vi "MIC_MD.vi"() -> ()   [LabVIEW 2012]
uses:
  GFG/GFGfpRefGet.vi
  GFG/GFGnumericGet.vi
  GFG/GFG library.lvlib
panel:
  out "Source VI":string
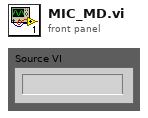
[diagram p1: front panel]
types:
  T1 = enum8{"Enabled", "Disabled", "Disabled and Grayed Out"}
  T2 = cluster{"WaveformChartRef":refnum<vi>, "DigitalRef":refnum<vi>, "ArrayRef":refnum<vi>, "TabControlRef":refnum<vi>, "EnumRef":refnum<vi>, "RingRef":refnum<vi>, "BooleanRef":refnum<vi>, "KnobRef":refnum<vi>, "SlideRef":refnum<vi>, "PathRef":refnum<vi>, "StringRef":refnum<vi>, "ComboBox":refnum<vi>, "WaveformGraphRef":refnum<vi>}
  T3 = enum16{"Left Button", "Center Button", "Right Button", "Window Close"}
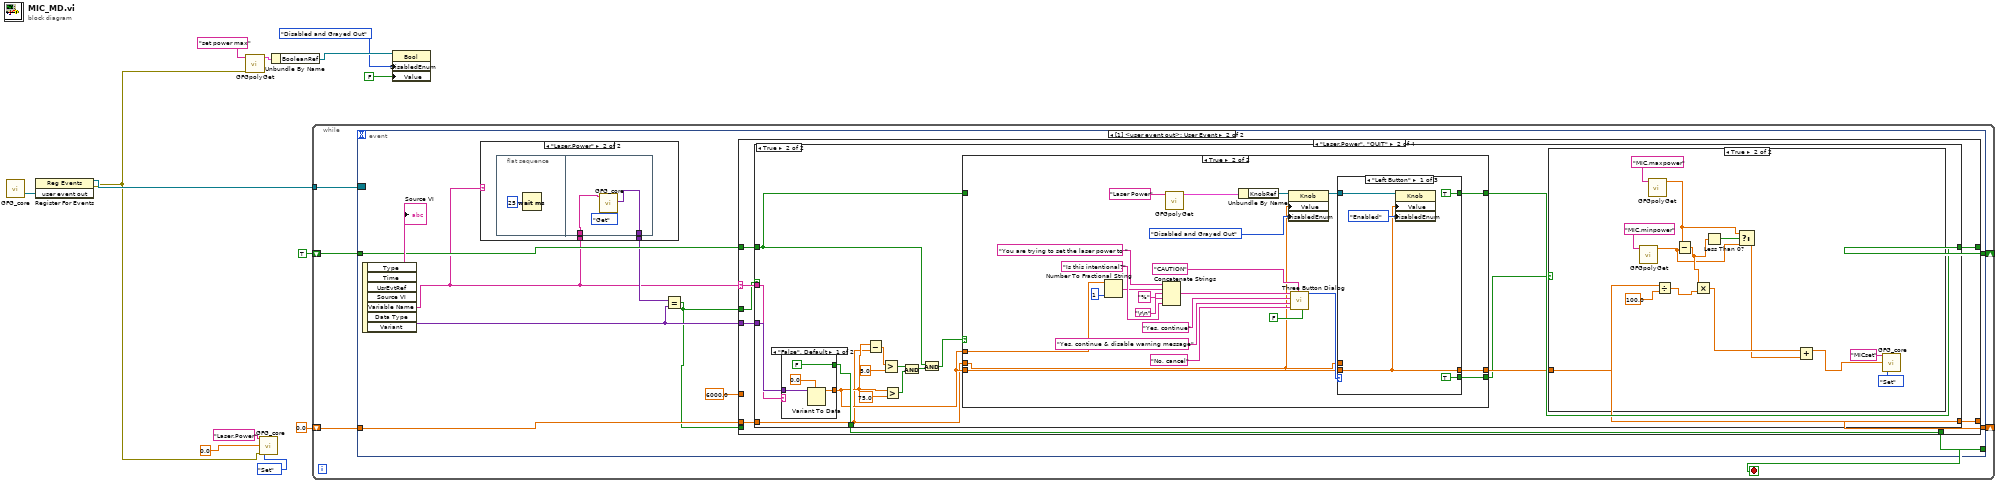
[diagram p0: block diagram]
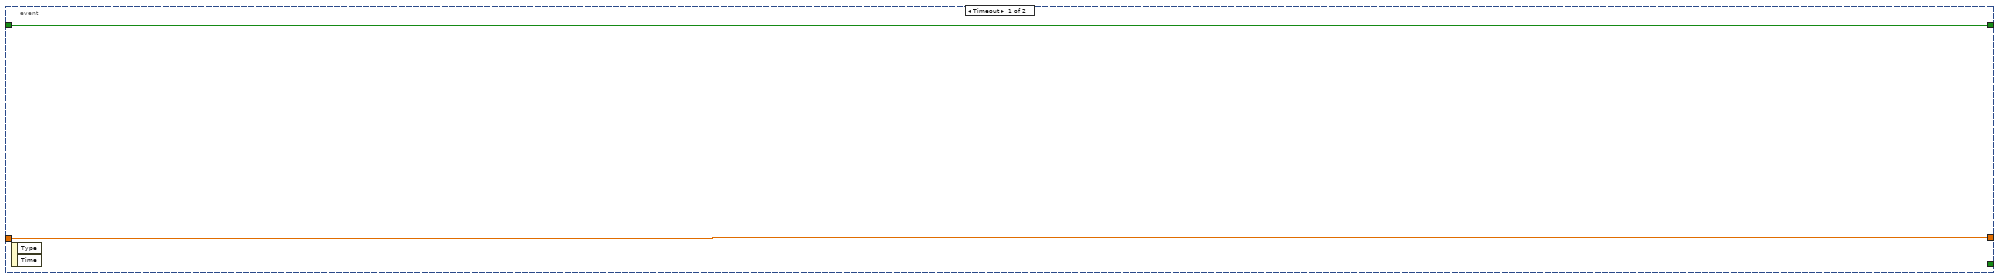
[diagram p2: hidden frame]
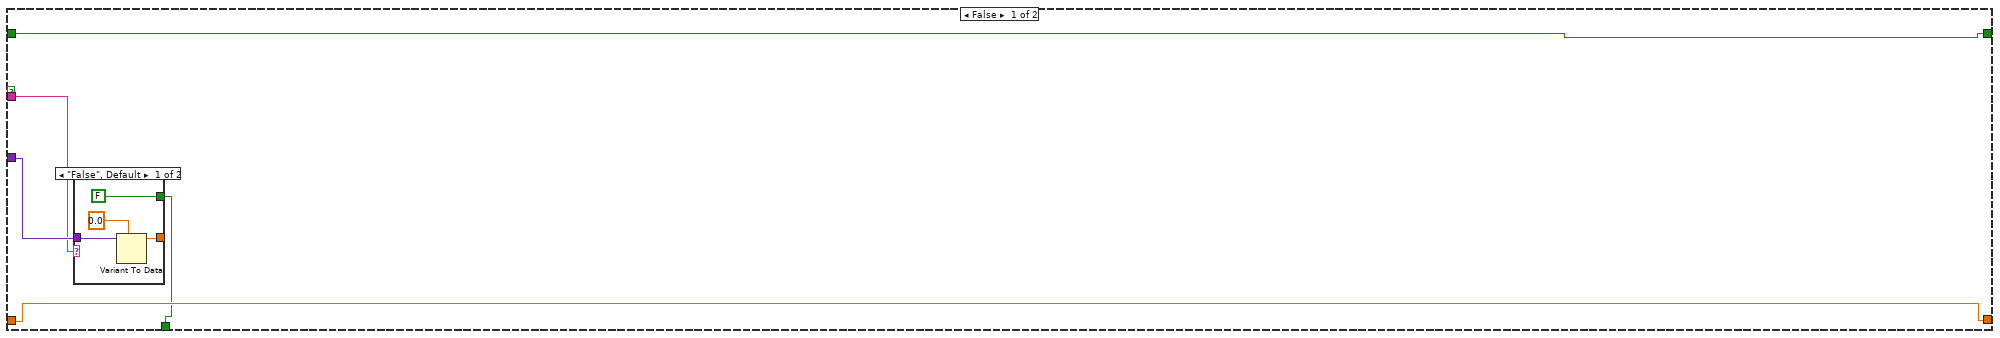
[diagram p5: hidden frame]
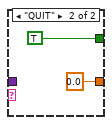
[diagram p6: hidden frame]
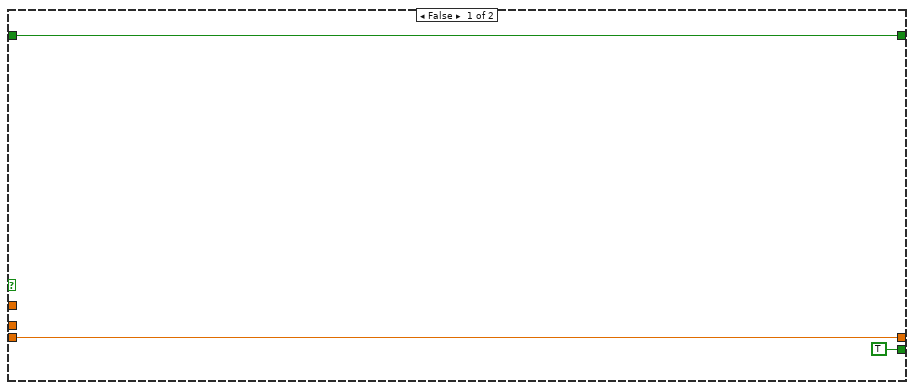
[diagram p8: hidden frame]
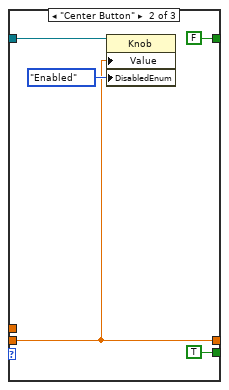
[diagram p9: hidden frame]
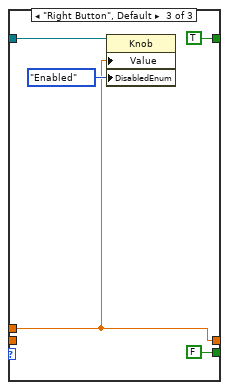
[diagram p10: hidden frame]
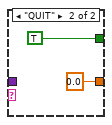
[diagram p11: hidden frame]
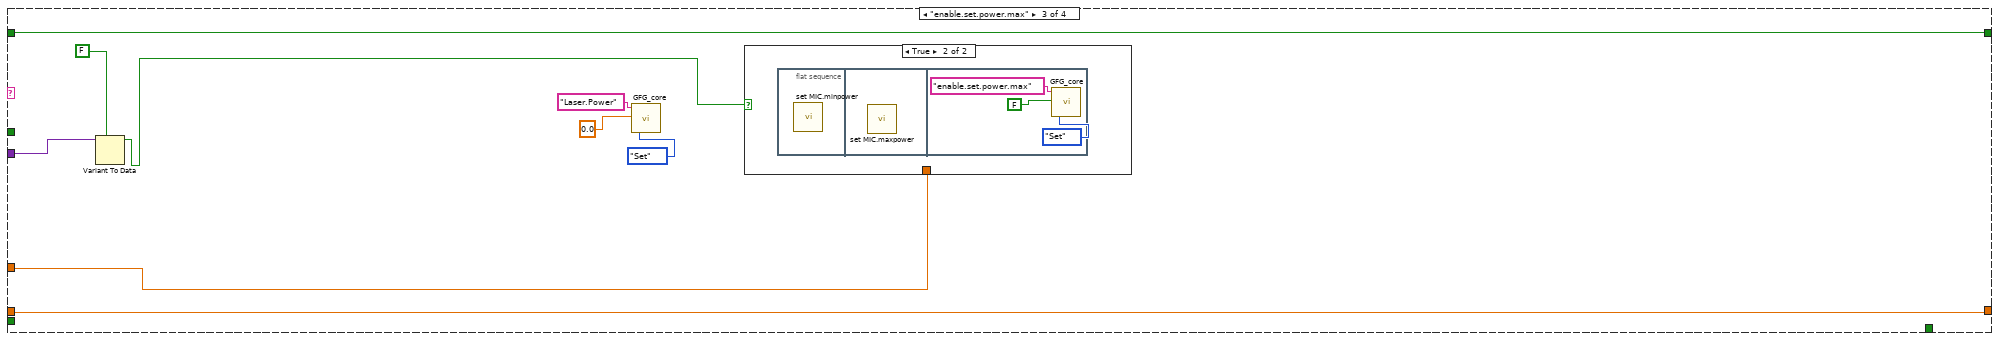
[diagram p12: hidden frame]
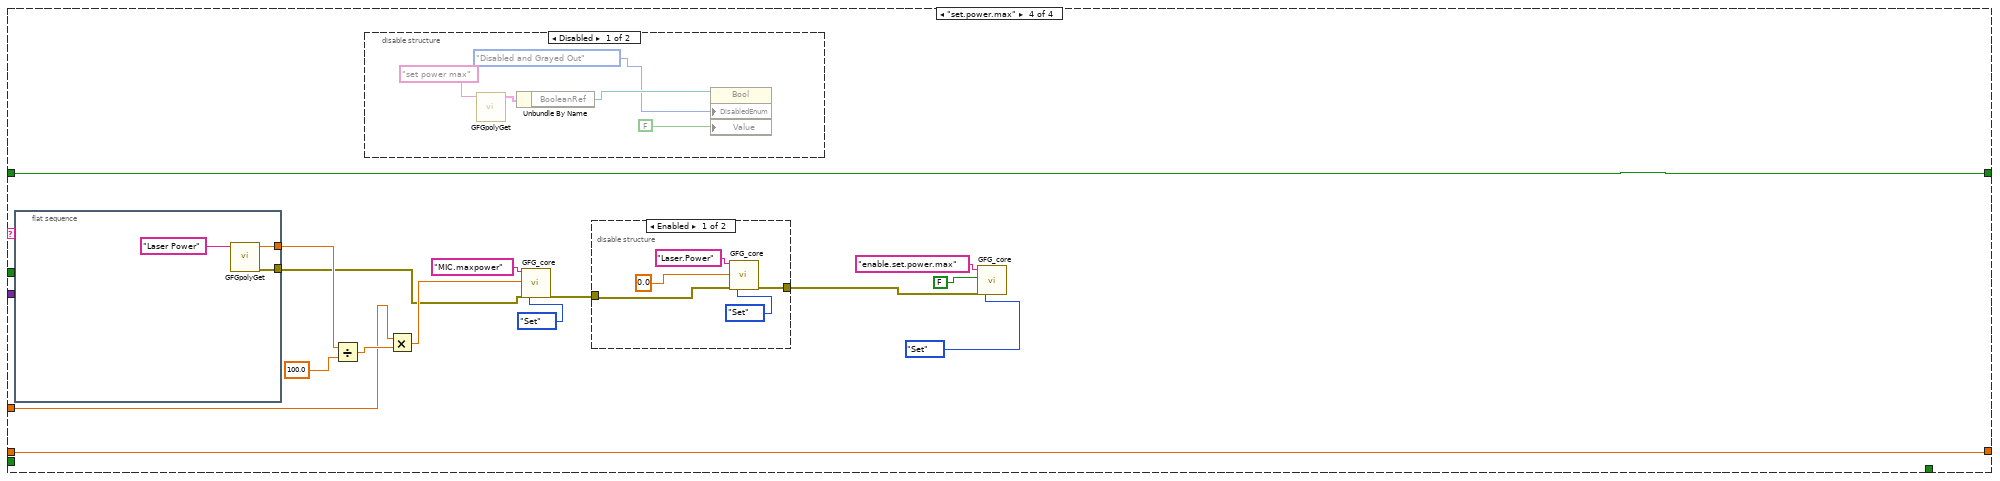
[diagram p14: hidden frame]
diagram:
  n1 = call "GFG_core.vi"() -> ("user event out"=w13:refnum<user-event>)  [unwired: 13 in, 6 out]
  n2 = register-events(w13) -> (reference out=w12:refnum<event-registration>, error out=w1:errorcluster)  [unwired: 2 in]
  n3 = call-poly "GFGpolyGet.vi"("error in (no error)"=w1, "Variable Name in"="set power max") -> ("output cluster"=w4:T2)  [unwired: 8 in, 1 out]
  n4 = call "GFG_core.vi"("Variable Name in"="Laser.Power", "Variant in"=0.0 ("Laser Power"), "error in (no error)"=w1, "Action"=enum16{"Init", "Set", "Get"}."Set") -> ()  [unwired: 9 in, 7 out]
  n5 = Unbundle By Name(w4) -> ("BooleanRef"=w5:refnum<vi>)
  n6 = while {
    tunnel: w12 -> [w19]
    shift-right: [w17] -> _
    shift-left: 0.0 ("Laser Power") -> [w16]
    shift-right: [w15] -> _
    shift-left: TRUE -> [w14]
    stop <- w18 stop-if-true
    n7 = event shown="[1] <user event out>: User Event" {
      selector: w19 -> [_ _]
      dyn-events: _ -> [_ _]
      timeout: _ -> [_ _]
      tunnel: [_ w31] -> w18
      tunnel: [w21 w30] -> w17
      tunnel: w16 -> [w21 w29]
      tunnel: [w20 w28] -> w15
      tunnel: w14 -> [w20 w27]
      event Timeout {
        n8 = event-data() -> ()  [unwired: 1 in, 2 out]
      }
      event User Event {
        n9 = event-data() -> ("Source VI"=→"Source VI":string, "Variable Name"=w22:string, "Variant"=w25:variant)  [unwired: 1 in, 4 out]
        n10 = case shown="\"Laser.Power\"" w22 {
          tunnel: w22 -> [w33 w35]
          tunnel: [w33 w34] -> w24
          frame "False", Default {
          }
          frame "Laser.Power" {
            n11 = flat-sequence {
              tunnel: w35 -> [w38]
              tunnel: [w37] -> w34
              frame #0 {
                n12 = Wait (ms)(milliseconds to wait=u32 25) -> ()  [unwired: 1 out]
              }
              frame #1 {
                n13 = call "GFG_core.vi"("Variable Name in"=w38, "Action"=enum16{"Init", "Set", "Get"}."Get") -> ("Variant Out"=w37:variant)  [unwired: 11 in, 6 out]
              }
            }
          }
        }
        n14 = Equal?(x=w24, y=w25) -> (x = y?=w23:bool)
        n15 = case shown="\"Laser.Power\", \"QUIT\"" w22 {
          selector: w22 -> [_ w48 _ _]
          tunnel: w25 -> [_ w49 w142 _]
          tunnel: [_ w47 _ _] -> w31
          tunnel: [w41 w44 w147 w165] -> w30
          tunnel: w29 -> [w41 w43 w147 w165]
          tunnel: [w40 w46 w146 w164] -> w28
          tunnel: w27 -> [w40 w45 w146 w164]
          tunnel: 6000.0 ("Laser Power") -> [_ _ w139 w151]
          tunnel: w23 -> [_ _ _ _]
          tunnel: w23 -> [_ w42 _ _]
          frame "False", Default {
          }
          frame "Laser.Power", "QUIT" {
            n16 = case shown="True" w42 {
              tunnel: w49 -> [w52 w76]
              tunnel: w48 -> [w51 w75]
              tunnel: [w50 w74] -> w47
              tunnel: [w53 w71] -> w46
              tunnel: w45 -> [w53 w69]
              tunnel: [w54 w68] -> w44
              tunnel: w43 -> [w54 w65]
              frame False {
                n17 = case shown="\"False\", Default" w51 {
                  tunnel: w52 -> [w58 _]
                  tunnel: [w57 0.0 ("Laser Power")] -> _
                  tunnel: [FALSE TRUE] -> w50
                  frame "False", Default {
                    n18 = Variant To Data(type=0.0 ("Laser Power"), Variant=w58) -> (data=w57:dbl)  [unwired: 1 in, 1 out]
                  }
                  frame "QUIT" {
                  }
                }
              }
              frame True {
                n19 = case shown="\"False\", Default" w75 {
                  tunnel: w76 -> [w136 _]
                  tunnel: [w135 0.0 ("Laser Power")] -> w66
                  tunnel: [FALSE TRUE] -> w74
                  frame "False", Default {
                    n20 = Variant To Data(type=0.0 ("Laser Power"), Variant=w136) -> (data=w135:dbl)  [unwired: 1 in, 1 out]
                  }
                  frame "QUIT" {
                  }
                }
                n21 = Subtract(x=w66, y=w65) -> (x-y=w64:dbl)
                n22 = Greater?(x=w64, y=5.0) -> (0:w62:bool)
                n23 = Greater?(x=w66, y=75.0) -> (0:w73:bool)
                n24 = And(x=w62, y=w73) -> (x .and. y?=w67:bool)
                n25 = And(x=w69, y=w67) -> (x .and. y?=w70:bool)
                n26 = case shown="True" w70 {
                  tunnel: [TRUE w111] -> w61
                  tunnel: [w92 w110] -> w71
                  tunnel: w69 -> [w92 _]
                  tunnel: w65 -> [_ w98]
                  tunnel: w66 -> [_ w108]
                  tunnel: w66 -> [w91 w99]
                  tunnel: [w91 w94] -> w68
                  frame False {
                  }
                  frame True {
                    n27 = Number To Fractional String(number=w108, precision (6)=i16 1) -> (F-format string=w97:string)  [unwired: 2 in]
                    n28 = Concatenate Strings("You are trying to set the laser power to " ("message"), w97, "%" ("string"), "\r\n", "Is this intentional?" ("string")) -> (w105:string)
                    n29 = call-poly "GFGpolyGet.vi"("Variable Name in"="Laser Power") -> ("output cluster"=w103:T2)  [unwired: 9 in, 1 out]
                    n30 = Unbundle By Name(w103) -> ("KnobRef"=w102:refnum<vi>)
                    n31 = property class="Knob"(reference=w102, "Value"=w98, "DisabledEnum"=T1."Disabled and Grayed Out" ("Disabled")) -> (reference out=w100:refnum<vi>)  [unwired: 1 in, 1 out]
                    n32 = call <vilib>:"Three Button Dialog.vi"("Allow user to close window? (TRUE)"=FALSE, "Window Title (\"\")"="CAUTION" ("Window Title (\"\")"), "Right Button Text (\"Cancel\")"="No, cancel" ("Right Button Text (\"Cancel\")"), "Center Button Text (\"No\")"="Yes, continue & disable warning message" ("Center Button Text (\"No\")"), "Left Button Text (\"Yes\")"="Yes, continue" ("Left Button Text (\"Yes\")"), "message"=w105) -> ("Which Button?"=w112:T3)  [unwired: 5 in]
                    n33 = case shown="\"Left Button\"" w112 {
                      tunnel: [TRUE TRUE FALSE] -> w111
                      tunnel: [TRUE FALSE TRUE] -> w110
                      tunnel: w100 -> [w119 w124 w129]
                      tunnel: w99 -> [w118 w123 _]
                      tunnel: w98 -> [_ _ w128]
                      tunnel: [w118 w123 w128] -> w94
                      frame "Left Button" {
                        n34 = property class="Knob"(reference=w119, "Value"=w118, "DisabledEnum"=T1."Enabled" ("Disabled")) -> ()  [unwired: 1 in, 2 out]
                      }
                      frame "Center Button" {
                        n35 = property class="Knob"(reference=w124, "Value"=w123, "DisabledEnum"=T1."Enabled" ("Disabled")) -> ()  [unwired: 1 in, 2 out]
                      }
                      frame "Right Button", Default {
                        n36 = property class="Knob"(reference=w129, "Value"=w128, "DisabledEnum"=T1."Enabled" ("Disabled")) -> ()  [unwired: 1 in, 2 out]
                      }
                    }
                  }
                }
                n37 = case shown="True" w61 {
                  tunnel: w68 -> [_ w87]
                  frame False {
                  }
                  frame True {
                    n38 = call-poly "GFGpolyGet.vi"("Variable Name in"="MIC.minpower") -> ("Numeric"=w79:dbl)  [unwired: 9 in, 1 out]
                    n39 = call-poly "GFGpolyGet.vi"("Variable Name in"="MIC.maxpower") -> ("Numeric"=w82:dbl)  [unwired: 9 in, 1 out]
                    n40 = Divide(x=w87, y=100.0 ("x")) -> (x/y=w90:dbl)
                    n41 = Subtract(x=w82, y=w79) -> (x-y=w84:dbl)
                    n42 = Multiply(x=w84, y=w90) -> (x*y=w88:dbl)
                    n43 = Less Than 0?(x=w84) -> (x < 0?=w83:bool)
                    n44 = Select(t=w82, s=w83, f=w79) -> (s? t:f=w80:dbl)
                    n45 = Add(x=w88, y=w80) -> (x+y=w81:dbl)
                    n46 = call "GFG_core.vi"("Variable Name in"="MICset", "Variant in"=w81, "Action"=enum16{"Init", "Set", "Get"}."Set") -> ()  [unwired: 10 in, 7 out]
                  }
                }
              }
            }
          }
          frame "enable.set.power.max" {
            n47 = Variant To Data(type=FALSE, Variant=w142) -> (data=w140:bool)  [unwired: 1 in, 1 out]
            n48 = call "GFG_core.vi"("Variable Name in"="Laser.Power", "Variant in"=0.0 ("Laser Power"), "Action"=enum16{"Init", "Set", "Get"}."Set") -> ()  [unwired: 10 in, 7 out]
            n49 = case shown="True" w140 {
              tunnel: w139 -> [_ _]
              frame False {
              }
              frame True {
                n50 = flat-sequence {
                  frame #0 {
                    n51 = call "set MIC.minpower.vi"() -> ()  [unwired: 12 in]
                  }
                  frame #1 {
                    n52 = call "set MIC.maxpower.vi"() -> ()  [unwired: 12 in]
                  }
                  frame #2 {
                    n53 = call "GFG_core.vi"("Variable Name in"="enable.set.power.max", "Variant in"=FALSE, "Action"=enum16{"Init", "Set", "Get"}."Set") -> ()  [unwired: 10 in, 7 out]
                  }
                }
              }
            }
          }
          frame "set.power.max" {
            n54 = flat-sequence {
              tunnel: [w172] -> w160
              tunnel: [w171] -> w157
              frame #0 {
                n55 = call-poly "GFGpolyGet.vi"("Variable Name in"="Laser Power") -> ("error out"=w171:errorcluster, "Numeric"=w172:dbl)  [unwired: 9 in]
              }
            }
            n56 = Divide(x=w160, y=100.0 ("x")) -> (x/y=w159:dbl)
            n57 = disable-structure shown="Disabled" {
              frame Disabled {
                n58 = call-poly "GFGpolyGet.vi"("Variable Name in"="set power max") -> ("output cluster"=w177:T2)  [unwired: 9 in, 1 out]
                n59 = Unbundle By Name(w177) -> ("BooleanRef"=w176:refnum<vi>)
                n60 = property class="Bool"(reference=w176, "DisabledEnum"=T1."Disabled and Grayed Out" ("Disabled"), "Value"=FALSE) -> ()  [unwired: 1 in, 2 out]
              }
              frame Enabled {
              }
            }
            n61 = Multiply(x=w151, y=w159) -> (x*y=w158:dbl)
            n62 = call "GFG_core.vi"("Variable Name in"="MIC.maxpower", "Variant in"=w158, "error in (no error)"=w157, "Action"=enum16{"Init", "Set", "Get"}."Set") -> ("error out"=w156:errorcluster)  [unwired: 9 in, 6 out]
            n63 = disable-structure shown="Enabled" {
              disable-tunnel: w156 -> [w167 _]
              disable-tunnel: [w166 _] -> w153
              frame Enabled {
                n64 = call "GFG_core.vi"("Variable Name in"="Laser.Power", "Variant in"=0.0 ("Laser Power"), "error in (no error)"=w167, "Action"=enum16{"Init", "Set", "Get"}."Set") -> ("error out"=w166:errorcluster)  [unwired: 9 in, 6 out]
              }
              frame Disabled {
              }
            }
            n65 = call "GFG_core.vi"("Variable Name in"="enable.set.power.max", "Variant in"=FALSE, "error in (no error)"=w153, "Action"=enum16{"Init", "Set", "Get"}."Set") -> ()  [unwired: 9 in, 7 out]
          }
        }
      }
    }
  }
  n66 = property class="Bool"(reference=w5, "DisabledEnum"=T1."Disabled and Grayed Out" ("Disabled"), "Value"=FALSE) -> ()  [unwired: 1 in, 2 out]
